vi "GEA2 Extract Message.vi"(8 "error in (no error)":errorcluster, 11 "GeaMessage":refnum<k24>) -> (0 "error out":errorcluster, 2 "Raw Data":string, 3 "GEA2 Data Out":T1 {"CRC" format="%04x"; "Length" format="%02x"; "Command" format="%02x"; "Destination" format="%02x"; "Source" format="%02x"})   [LabVIEW 2016, in "GEA2_Toolkit.lvlib"]
uses:
  library/GEA2_Toolkit.lvlib
  C:/Technology Lab/NI-2010/Trunk/Utility/LabVIEW GEA2 Toolkit v1.0.0.0/Appliance.NET/GeaCommunication.dll
  Appliance.NET/GeaCommunication.dll
  type defs/Data Out.ctl
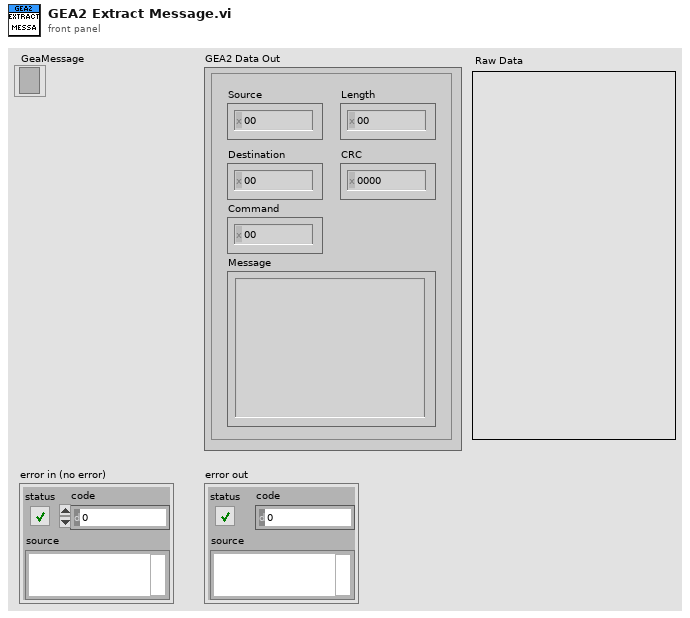
[diagram p1: front panel]
types:
  T1 = typedef "GEA2_Toolkit.lvlib/Data Out.ctl" = cluster{"Source":u8, "Destination":u8, "Command":u8, "Length":u8, "CRC":u16, "Message":string}
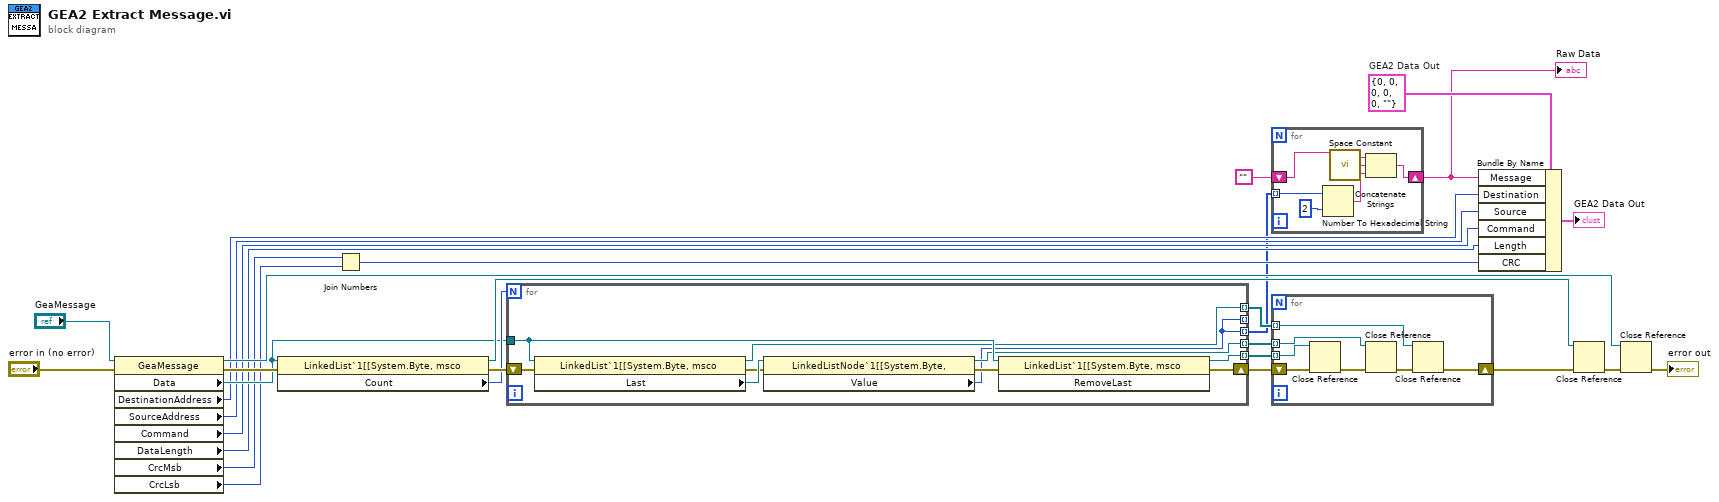
[diagram p0: block diagram]
diagram:
  w4 = T1 {"Source"=0, "Destination"=0, "Command"=0, "Length"=0, "CRC"=0, "Message"=""}  # GEA2 Data Out
  n1 = property class="GeaMessage"(reference="GeaMessage", error in="error in (no error)") -> (reference out=w22:refnum<k24>, error out=w23:errorcluster, "Data"=w15:refnum<k24>, "DestinationAddress"=w5:u8, "SourceAddress"=w6:u8, "Command"=w7:u8, "DataLength"=w10:u8, "CrcMsb"=w12:u8, "CrcLsb"=w13:u8)
  n2 = property class="LinkedList`1[[System.Byte, msco"(reference=w15, error in=w23) -> (reference out=w21:refnum<k24>, error out=w24:errorcluster, "Count"=w16:i32)
  n3 = Join Numbers(hi=w12, lo=w13) -> ((hi.lo)=w14:u16)
  n4 = for {
    N: w16 -> [_]
    tunnel: [w28] -> _ mode=indexing
    shift-right: [w33] -> w25
    shift-left: w24 -> [w36]
    tunnel: w15 -> [w32]
    tunnel: [w31] -> w18 mode=indexing
    tunnel: [w30] -> w19 mode=indexing
    tunnel: [w29] -> w17 mode=indexing
    tunnel: [w28] -> w3 mode=indexing
    n5 = property class="LinkedList`1[[System.Byte, msco"(reference=w32, error in=w36) -> (reference out=w29:refnum<k24>, error out=w35:errorcluster, "Last"=w37:refnum<k24>)
    n6 = property class="LinkedListNode`1[[System.Byte, "(reference=w37, error in=w35) -> (reference out=w31:refnum<k24>, error out=w34:errorcluster, "Value"=w28:u8)
    n7 = invoke class="LinkedList`1[[System.Byte, msco" method="RemoveLast"(reference=w32, error in=w34) -> (reference out=w30:refnum<k24>, error out=w33:errorcluster)  [unwired: 1 in, 1 out]
  }
  n8 = for {
    tunnel: w3 -> [w43] mode=indexing
    shift-right: [w42] -> w1
    shift-left: "" -> [w41]
    n9 = Number To Hexadecimal String(1:i16 2 ("width (-)"), 2:w43) -> (0:w39:string)
    n10 = call <vilib>:"Space Constant.vi"() -> ("String"=w38:string)
    n11 = Concatenate Strings(w41, w38, w39) -> (w42:string)
  }
  "Raw Data" <- w1
  n12 = for {
    tunnel: w19 -> [w50] mode=indexing
    tunnel: w18 -> [w49] mode=indexing
    shift-right: [w45] -> w20
    shift-left: w25 -> [w48]
    tunnel: w17 -> [w44] mode=indexing
    n13 = Close Reference(reference=w50, error in (no error)=w48) -> (error out=w47:errorcluster)
    n14 = Close Reference(reference=w49, error in (no error)=w47) -> (error out=w46:errorcluster)
    n15 = Close Reference(reference=w44, error in (no error)=w46) -> (error out=w45:errorcluster)
  }
  n16 = Bundle By Name(cluster=w4, "Message"=w1, "Destination"=w5, "Source"=w6, "Command"=w7, "Length"=w10, "CRC"=w14) -> (→"GEA2 Data Out":T1)
  n17 = Close Reference(reference=w21, error in (no error)=w20) -> (error out=w27:errorcluster)
  n18 = Close Reference(reference=w22, error in (no error)=w27) -> (error out=→"error out":errorcluster)
